vi "DeCoF binary to float array.vi"(1 "byte buffer":u8[](array[numeric])) -> (0 "float array":sgl[](array[numeric]))   [LabVIEW 2013]
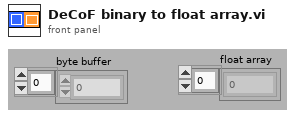
[diagram p1: front panel]
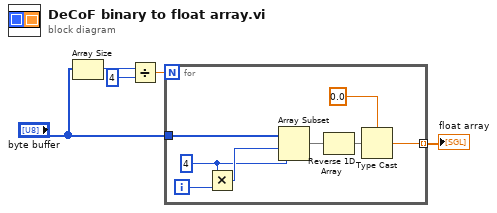
[diagram p0: block diagram]
diagram:
  n1 = Array Size(array="byte buffer") -> (size(s)=w5:i32)
  n2 = Divide(x=w5, y=4) -> (x/y=w2:dbl)
  n3 = for {
    N: w2 -> [_]
    tunnel: "byte buffer" -> [w12]
    tunnel: [w6] -> w3 mode=indexing
    i -> [w13]
    w10 = 4 ("x")
    n4 = Multiply(x=w10, y=w13) -> (x*y=w11:i32)
    n5 = Array Subset(array=w12, index=w11, length=w10) -> (w9:u8[])
    n6 = Reverse 1D Array(array=w9) -> (reversed array=w8:u8[])
    n7 = Type Cast(type=sgl 0.0, x=w8) -> (*(type *) &x=w6:sgl)
  }
  "float array" <- w3
